vi "Main.vi"   [LabVIEW 2017, in "BridgePatternDemo.lvclass"]
uses:
  BridgePatternDemo.lvclass
  Tv Class/Tv.lvclass
  C:/Users/fflores/Documents/LabVIEW-Open-Projects/LabIVEW OOP Design Patterns/Bridge Pattern/Device Class/Device.lvclass
  Radio Class/Radio.lvclass
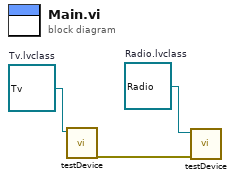
[diagram p0: block diagram]
diagram:
  w2 = refnum<class "Radio.lvclass"> refnum  # Radio.lvclass
  w3 = refnum<class "Tv.lvclass"> refnum  # Tv.lvclass
  n1 = call "testDevice.vi"("Device.lvclass"=w3) -> ("error out"=w1:errorcluster)  [unwired: 10 in]
  n2 = call "testDevice.vi"("error in (no error)"=w1, "Device.lvclass"=w2) -> ()  [unwired: 9 in, 1 out]
